vi "Multi Instrument Do Core.vi"(8 "error in (no error)":errorcluster, 10 "Actor in":refnum<class "Actor.lvclass">, 11 "Instrument Msg in":refnum<class "Test Nested Multi Instrument Msg.lvclass">) -> (0 "error out":errorcluster, 1 "Data":refnum<class "Data.lvclass">, 2 "Actor out":refnum<class "Actor.lvclass">, 3 "Instrument Msg out":refnum<class "Test Nested Multi Instrument Msg.lvclass">)   [LabVIEW 2020, in "Test.lvlib" / "Test Nested Multi Instrument Msg.lvclass"]
doc: "Message interaction with multiple instruments is handled by the Multi Instrument Do Core.\n\nMulti Instrument Msgs contains the Cores of all the Owners they require. Keep this in mind if the message wire is branched. Incorrect synchronization of nested Multi Instrument Msgs can lead to deadlocks if wire branching is used incorrectly!\n\nThe default implementation does nothing."
uses:
  Test Nested Multi Instrument Msg.lvclass
  PPL/HDH.Actor Framework.Core.Actor.lvlibp/1abvi3w/vi.lib/ActorFramework/Actor/Actor.lvclass
  PPL/HDH.Data.Generic.lvlibp/Data.lvclass
  Test Multi Instrument Msg/Test Multi Instrument Msg.lvclass
  PPL/HDH.Actor Framework.Core.Instrument Handler.lvlibp/Messages/Multi Instrument Msg/Multi Instrument Msg.lvclass
  C:/Current projects/WS/PPL/HDH.Actor Framework.Core.Instrument Handler.lvlibp/Messages/Instrument Msg/Instrument Msg.lvclass
  C:/Current projects/WS/PPL/HDH.Actor Framework.Core.Instrument Handler.lvlibp/Messages/Multi Instrument Msg/Multi Instrument Msg.lvclass
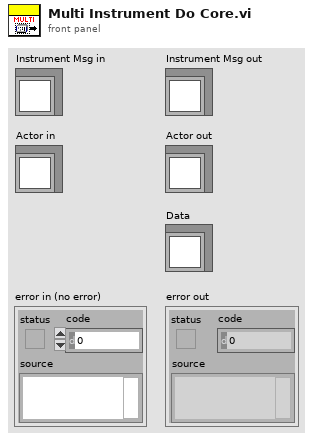
[diagram p1: front panel]
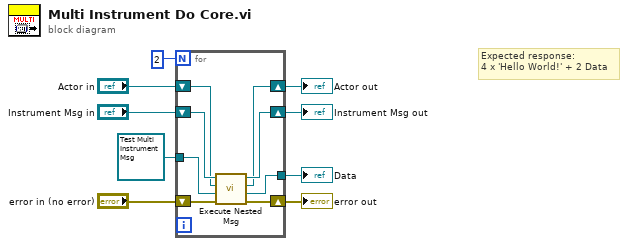
[diagram p0: block diagram]
diagram:
  # "Expected response:\n4 x 'Hello World!' + 2 Data"
  n1 = for {
    N: 2 -> [_]
    tunnel: refnum<class "Test Multi Instrument Msg.lvclass"> refnum ("Test.lvlib:Test Multi Instrument Msg.lvclass") -> [w16]
    tunnel: [w11] -> w4
    shift-right: [w10] -> w3
    shift-left: "error in (no error)" -> [w17]
    shift-right: [w14] -> w7
    shift-left: "Instrument Msg in" -> [w15]
    shift-right: [w12] -> w5
    shift-left: "Actor in" -> [w13]
    n2 = call "Execute Nested Msg.vi"("error in (no error)"=w17, "Instrument Msg to Run"=w16, "Actor in"=w13, "Multi Instrument Msg in"=w15) -> ("error out"=w10:errorcluster, "Data"=w11:refnum<class "Data.lvclass">, "Actor out"=w12:refnum<class "Actor.lvclass">, "Multi Instrument Msg out"=w14:refnum<class "Test Nested Multi Instrument Msg.lvclass">)  [unwired: 3 in, 1 out]
  }
  "error out" <- w3
  "Instrument Msg out" <- w7
  "Actor out" <- w5
  "Data" <- w4
